vi "TC560-Error Handle.vi"(8 "error in":errorcluster, 11 "Respond In":string) -> (0 "error out":errorcluster, 3 "Respond Out":string)   [LabVIEW 2018]
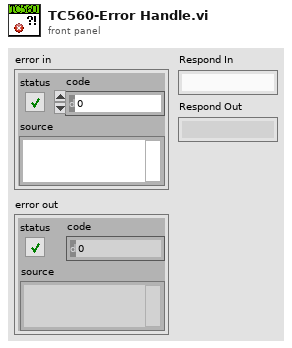
[diagram p1: front panel]
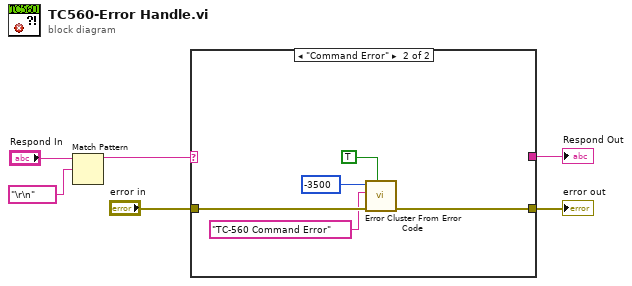
[diagram p0: block diagram]
diagram:
  n1 = Match Pattern(string="Respond In", regular expression="\r\n" ("write buffer")) -> (before substring=w1:string)  [unwired: 1 in, 3 out]
  n2 = case shown="\"Command Error\"" w1 {
    selector: w1 -> [w8 _]
    tunnel: "error in" -> [w7 w13]
    tunnel: [w7 w12] -> w5
    tunnel: [w8 _] -> w4
    frame Default {
    }
    frame "Command Error" {
      n3 = call <vilib>:"Error Cluster From Error Code.vi"("show call chain? (False)"=TRUE, "error in (no error)"=w13, "error message (\"\")"="TC-560 Command Error" ("error message (\"\")"), "error code (0)"=-3500) -> ("error out"=w12:errorcluster)  [unwired: 5 in]
    }
  }
  "error out" <- w5
  "Respond Out" <- w4
